vi "Get Project Tasks.vi"(8 "error in (no error)":errorcluster, 10 "Project Name":string, 11 "Projects in":refnum<class "Projects.lvclass">) -> (0 "error out":errorcluster, 2 "Tasks":string[](array[string]), 3 "Projects out":refnum<class "Projects.lvclass">)   [LabVIEW 2020, in "Projects.lvclass"]
doc: "Reads the tasks from the Map for the indicated Project Name. If no tasks are present or the project name is not present in the Map data then the Tasks output will be an empty array.\n\n03/2025 Erich Schlieper"
uses:
  Projects.lvclass
  Projects.lvclass/Projects.ctl
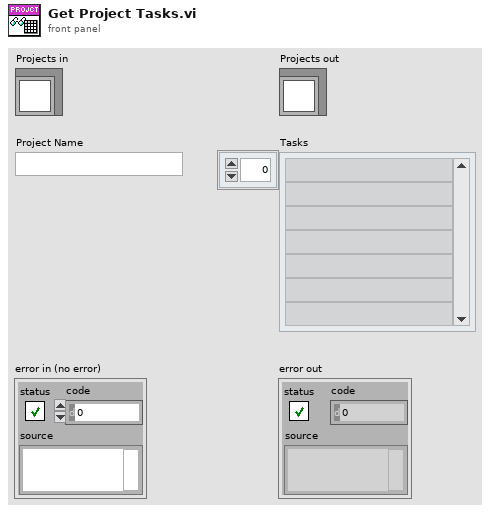
[diagram p1: front panel]
types:
  T1 = typedef "Project Info.ctl" = cluster{"Project Active?":bool, "Tasks":set{string}, "Task Active":map{string, bool}}
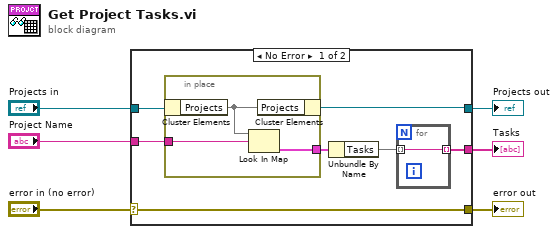
[diagram p0: block diagram]
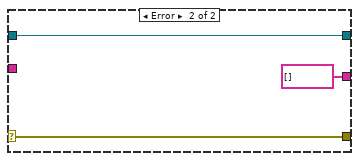
[diagram p2: hidden frame]
diagram:
  n1 = case shown="No Error" "error in (no error)" {
    selector: "error in (no error)" -> [w12 w20]
    tunnel: [w12 w20] -> w5
    tunnel: [w11 w19] -> w3
    tunnel: "Projects in" -> [w13 w19]
    tunnel: "Project Name" -> [w10 _]
    tunnel: [w8 string[] []] -> w1
    frame No Error {
      n2 = in-place {
        in-place-border: w10 -> [w15]
        in-place-border: [w14] -> w9
        n3 = in-place-cluster #1(w13) -> ("Projects"=w16:map{string, T1})
        n4 = Look In Map(map=w16, key=w15) -> (value=w14:T1)  [unwired: 1 in, 1 out]
        n5 = in-place-cluster #1("Projects"=w16) -> (w11:refnum<class "Projects.lvclass">)
      }
      n6 = Unbundle By Name(w9) -> ("Tasks"=w7:set{string})
      n7 = for {
        tunnel: [w17] -> w8 mode=indexing
        tunnel: w7 -> [w17] mode=indexing
      }
    }
    frame Error {
    }
  }
  "error out" <- w5
  "Projects out" <- w3
  "Tasks" <- w1
